vi "State Enqueue.vi"(8 "error in (no error)":errorcluster, 9 "Display State Change Class":T1, 11 "Control Ref Queue":T2) -> (0 "error out":errorcluster)   [LabVIEW 2017, in "3D Plot.lvclass"]
uses:
  <vilib>/Math Plots/3D Math Plots/3D Plot/3D Plot/3D Plot.lvclass
  <vilib>/Math Plots/3D Math Plots/3D Plot/Action String/3DMathPlot Ctrl Act Queue.ctl
  <vilib>/Math Plots/3D Math Plots/3D Plot/Action String/3DMathPlot Ctrl Act Cluster.ctl
  <vilib>/Math Plots/3D Math Plots/3D Plot/Action String/3DMathPlot State Class.ctl
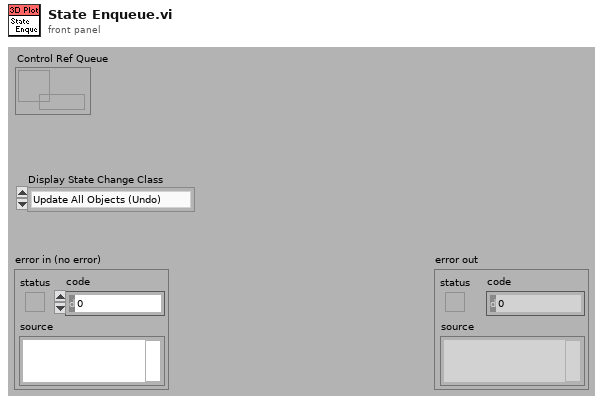
[diagram p1: front panel]
types:
  T1 = typedef "3DMathPlot State Class.ctl" = enum16{"Update All Objects (Undo)", "Update Light Object Only", "Update Axis Object Only", "Update Plot Object Only", "Update Cursor Object Only", "Update Axis Plot Cursor Objects", "No Update"}
  T2 = typedef "3DMathPlot Ctrl Act Queue.ctl" = refnum<queue>
  T3 = typedef "3DMathPlot Ctrl Act Cluster.ctl" = cluster{"3D Picture Control":refnum<vi>, "Render Window Refnum":refnum<vi>, "XY Graph":refnum<vi>, "Intensity Graph":refnum<vi>, "Color Legend Palette":refnum<vi>, "Projection Palette":refnum<vi>, "XControl  Ref":refnum<vi>, "Facade Ref":refnum<vi>, "Export Image Ref":refnum<vi>, "Clear Data Flag":bool, "Display State Change Class":T1}
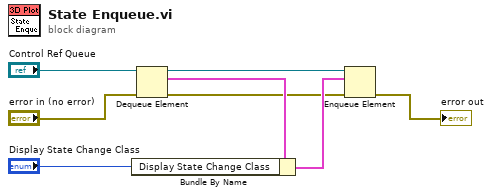
[diagram p0: block diagram]
diagram:
  n1 = Dequeue Element(queue="Control Ref Queue", error in (no error)="error in (no error)") -> (queue out=w7:T2, element=w6:T3, error out=w3:errorcluster)  [unwired: 2 out]
  n2 = Bundle By Name(cluster=w6, "Display State Change Class"="Display State Change Class") -> (w4:T3)
  n3 = Enqueue Element(queue=w7, element=w4, error in (no error)=w3) -> (error out=→"error out":errorcluster)  [unwired: 3 out]
